vi "Set Step Name.vi"(8 "error in (no error)":errorcluster, 10 "Step In":refnum<k7>, 11 "NULL_ADAPTER in":refnum<class "Null Adapter.lvclass">) -> (0 "error out":errorcluster, 2 "Step Out":refnum<k7>, 3 "NULL_ADAPTER out":refnum<class "Null Adapter.lvclass">)   [LabVIEW 2018, in "Null Adapter.lvlib" / "Null Adapter.lvclass"]
uses:
  Null Adapter.lvclass
  c:/Sequence Automation/Plugins/Measurement Interface.lvlibp/Measurement Interface.lvclass
  Plugins/Measurement Interface.lvlibp/Private Methods/Measurement Name/Read Measurement Name.vi
  Plugins/TestStand API Tools (TSAT).lvlibp/Step Actions/TSAT Step Actions.lvlib
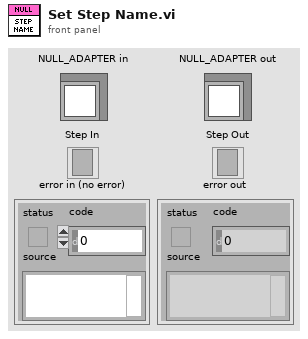
[diagram p1: front panel]
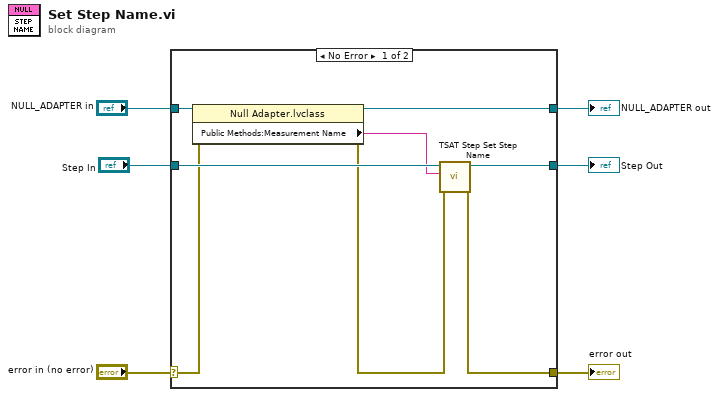
[diagram p0: block diagram]
diagram:
  n1 = case shown="No Error" "error in (no error)" {
    selector: "error in (no error)" -> [w10 w17]
    tunnel: [w8 w17] -> w5
    tunnel: [w13 w16] -> w3
    tunnel: "NULL_ADAPTER in" -> [w14 w16]
    tunnel: "Step In" -> [w12 w15]
    tunnel: [w11 w15] -> w1
    frame No Error {
      n2 = property class="Null Adapter.lvclass"(reference=w14, error in=w10) -> (reference out=w13:refnum<class "Null Adapter.lvclass">, error out=w9:errorcluster, "Public Methods:Measurement Name"=w7:string)
      n3 = call "TSAT Step Set Step Name.vi"("Error In"=w9, "Name"=w7, "Step In"=w12) -> ("Error Out"=w8:errorcluster, "Step Out"=w11:refnum<k7>)  [unwired: 7 in]
    }
    frame Error {
    }
  }
  "error out" <- w5
  "NULL_ADAPTER out" <- w3
  "Step Out" <- w1
